vi "Process.vi"(8 "error in":errorcluster, 11 "Inst.Xeryon-Rotator":refnum<class "Inst.Xeryon-Rotator.lvclass">) -> (0 "error out":errorcluster, 3 "Inst.Xeryon-Rotator out":refnum<class "Inst.Xeryon-Rotator.lvclass">)   [LabVIEW 2019, in "Inst.Xeryon-Rotator.lvclass"]
doc: "---------------------------------------------------------------\nJKI State Machine Objects™\nhttp://jki.net/state-machine-objects/\nCopyright (C) 2005-2015, JKI <info@jki.net>\nALL RIGHTS RESERVED"
uses:
  Inst.Xeryon-Rotator.lvclass
  C:/Program Files (x86)/National Instruments/LabVIEW 2019/vi.lib/JKI/JKI SMO/SMO/SMO.lvclass
  C:/Program Files (x86)/National Instruments/LabVIEW 2019/user.lib/LevyLab/Instrument Framework/Instrument/Instrument.lvclass
  Typedefs/PrivateEvents--Inst.Xeryon-Rotator.MessageToProcess.ctl
  <userlib>/LevyLab/RemoteControl/RemoteControl/Typedefs/Message--Cluster.ctl
  <vilib>/JKI/JKI SMO/SMO/SMO.lvclass/SMO.ctl
  Inst.Xeryon-Rotator.lvclass/Inst.Xeryon-Rotator.ctl
  <userlib>/LevyLab/Instrument Framework/Instrument Types/Cryostat/Typedefs/setAngle--cluster.ctl
  Typedefs/Inst.Xeryon-Rotator.ScanState--Enum.ctl
  cbce47eb-2e04-4774-9aae-1c3eb2914706.vi
  f3e0a8c3-f545-4415-8120-73ea4d9772d3.vi
  828899be-930a-4dca-b584-bfe75166f4b0.vi
  bd7500a4-fca6-4b1e-8595-4df63a7e1bab.vi
  <vilib>/JKI/JKI SMO/SMO/Private/ReftoDVR--SMO.vi
  f3e0a8c3-f545-4415-8120-73ea4d9772d3.vi/fb9ef9f7-99d0-4ee5-81e5-6076cd542a2f.vi
  f3e0a8c3-f545-4415-8120-73ea4d9772d3.vi/df923573-e8f3-4648-a92f-bb60dda59a34.vi
  828899be-930a-4dca-b584-bfe75166f4b0.vi/24a7be02-affa-44f0-9bee-c77722484ac6.vi
  828899be-930a-4dca-b584-bfe75166f4b0.vi/9b5d2591-8431-4617-9ceb-7f0da0949f44.vi
  bd7500a4-fca6-4b1e-8595-4df63a7e1bab.vi/1d6531ba-9a80-485c-81e6-b1433e72d2e7.vi
  bd7500a4-fca6-4b1e-8595-4df63a7e1bab.vi/5f7f602e-e2b4-4f16-b1e8-66f0979bfccf.vi
  <vilib>/JDP Science/JSONtext/Variant to JSON Text.vi
  <vilib>/Utility/Data Type/Get Type Information.vi
  <vilib>/JDP Science/JSONtext/JSON text to Variant.vi
  <vilib>/JDP Science/JSONtext/LVClass Serializer/JSONtext LVClass Serializer.lvclass
  <userlib>/LevyLab/Instrument Framework/Instrument Types/Cryostat/Instrument.Cryostat.lvclass
  <userlib>/LevyLab/Instrument Framework/Instrument/Instrument.lvclass
  <userlib>/LevyLab/RemoteControl/RemoteControl/RemoteControl.lvclass
  <vilib>/JDP Science/JSONtext/JSONtext.lvlib
  <userlib>/LevyLab/Debug/Debug.lvlib
  <userlib>/LevyLab/Instrument Framework/Instrument/API/Instrument.sendMessageToProcess (variant).vi
  <vilib>/JKI/JKI SMO/SMO/SMO.lvclass
panel:
  out "Data":string
  out "Status":string
  out "State History":string
  # "Instrument.Xeryon-Rotator"
  # "Xeryon-Rotator"
  # "For instructions on how to use the JKI State Machine Objects, examples and video tutorials, visit:\nhttp://jki.net/state-machine-objects/\n\nJKI State Machine Objects™\nhttp://jki.net/state-machine-objects/\nCopyright (C) 2005-2015, JKI <info@jki.net>\nALL RIGHTS RESERVED"
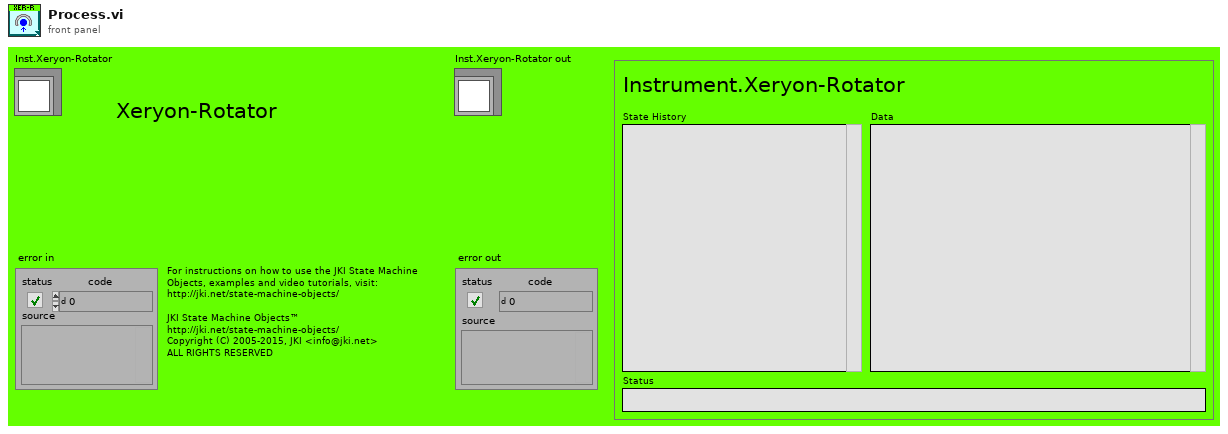
[diagram p1: front panel]
types:
  T1 = enum32{"invalid app kind", "Development System", "Run Time System", "Student Edition", "Embedded LabVIEW", "Evaluation", "Custom"}
  T2 = enum32{"Invalid", "Standard", "Closed", "Hidden", "Minimized", "Maximized"}
  T3 = typedef "Instrument.Cryostat.lvclass/setAngle--cluster.ctl" = cluster{"angle":dbl, "rate":dbl, "channel":i32}
  T4 = typedef "Inst.Xeryon-Rotator.lvclass/Inst.Xeryon-Rotator.ScanState--Enum.ctl" = enum16{"Scan Left", "Stop", "Scan Right", "Reset"}
  T5 = typedef "RemoteControl.lvlib/RemoteControl.lvclass/Message--Cluster.ctl" = cluster{"Command":string, "Data":variant, "ID":string, "error":errorcluster}
  T6 = typedef "Inst.Xeryon-Rotator.lvclass/PrivateEvents--Inst.Xeryon-Rotator.MessageToProcess.ctl" = cluster{"Message":T5}
  T7 = cluster{"Core":cluster{"Current VI Reference":refnum<vi>, "Close Panel on Exit?":bool, "Last Error":cluster{"error":errorcluster, "previous state":string, "remaining states":string}, "Shutdown?":bool}, "SelfRef":refnum<class "Inst.Xeryon-Rotator.lvclass">, "Running Step":i32, "sequence":string[], "MessageToProcess":T6}
  T8 = cluster{"Current VI Reference":refnum<vi>, "Close Panel on Exit?":bool, "Last Error":cluster{"error":errorcluster, "previous state":string, "remaining states":string}, "Shutdown?":bool}
  T9 = typedef "Debug.lvlib/Attribute.Debug.lvclass/DebugBehavior.ctl" = enum16{"Normal", "Debug"}
  T10 = typedef "SMO.lvclass/Protected Events.ctl" = cluster{"StopProcesses":refnum<user-event>, "AbortProcesses":refnum<user-event>, "Config Changed":refnum<user-event>, "Dependency":refnum<user-event>}
  T11 = cluster{"Encoder position [selected units]":dbl, "Desired Position [selected units]":dbl, "Status":string}
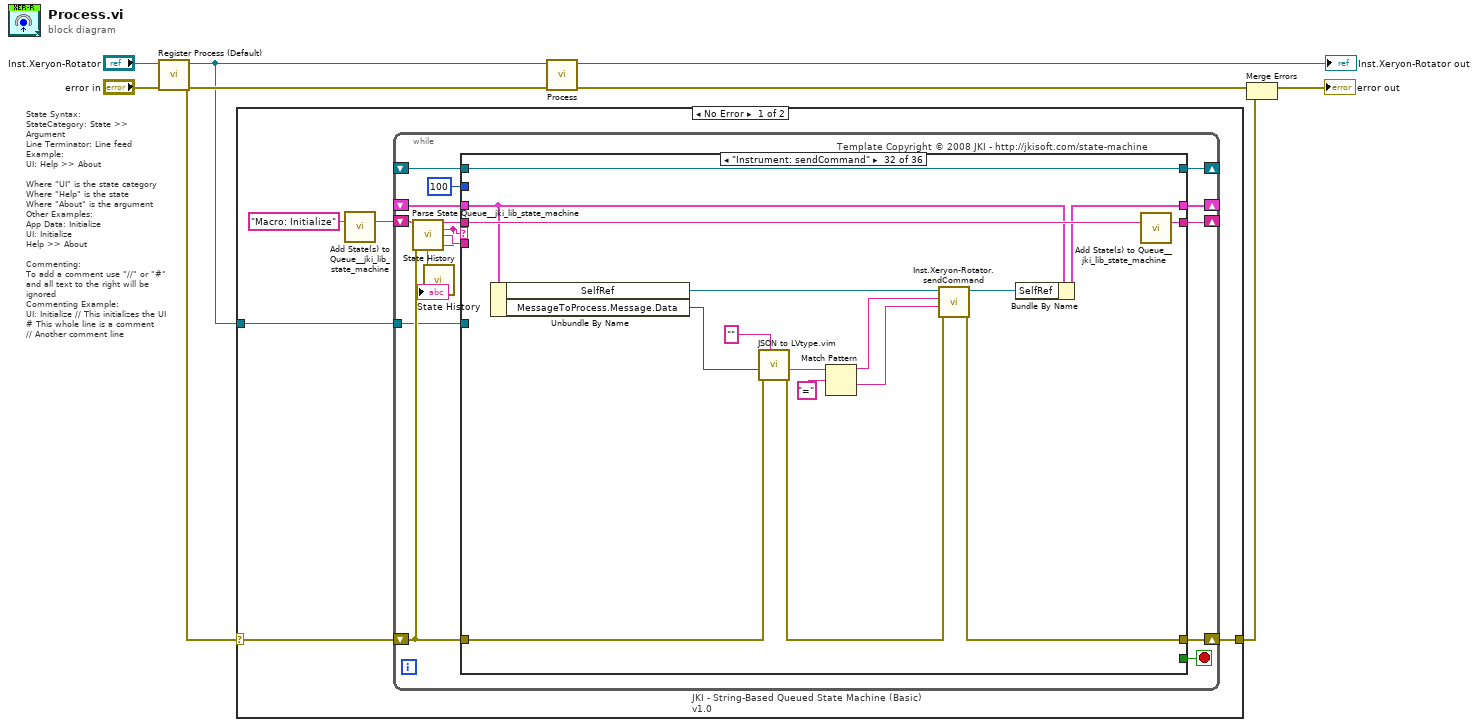
[diagram p0: block diagram]
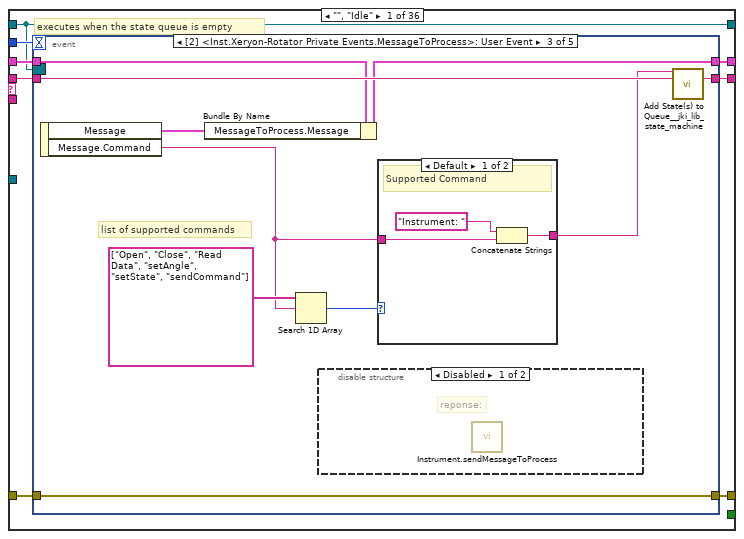
[diagram p2: hidden frame]
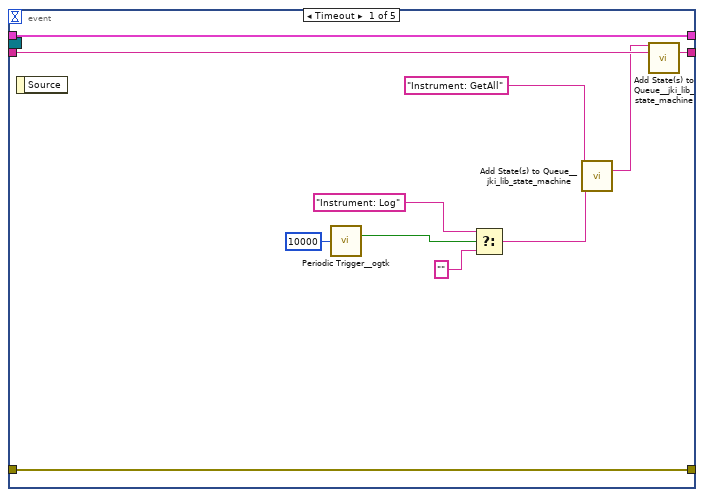
[diagram p3: hidden frame]
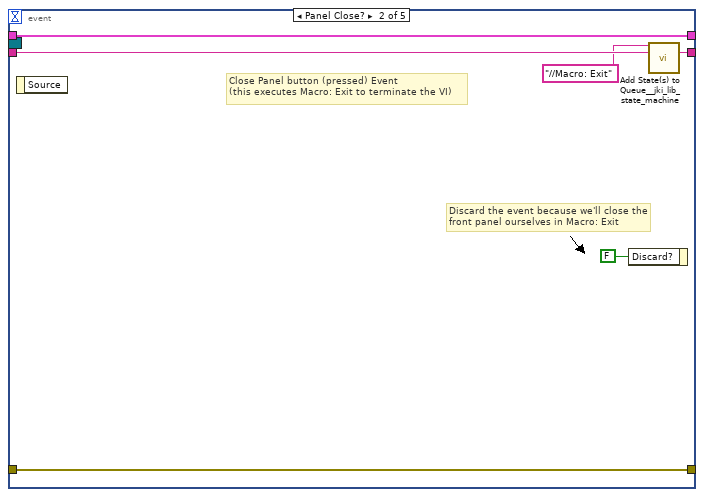
[diagram p4: hidden frame]
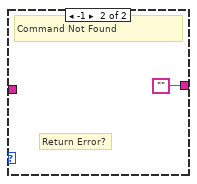
[diagram p6: hidden frame]
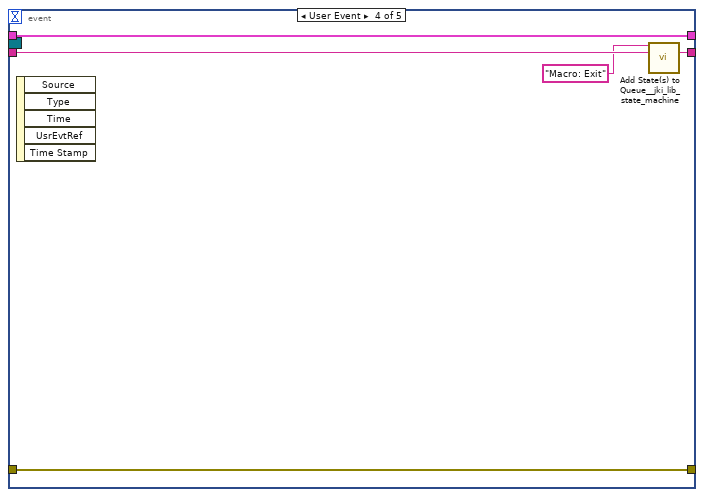
[diagram p7: hidden frame]
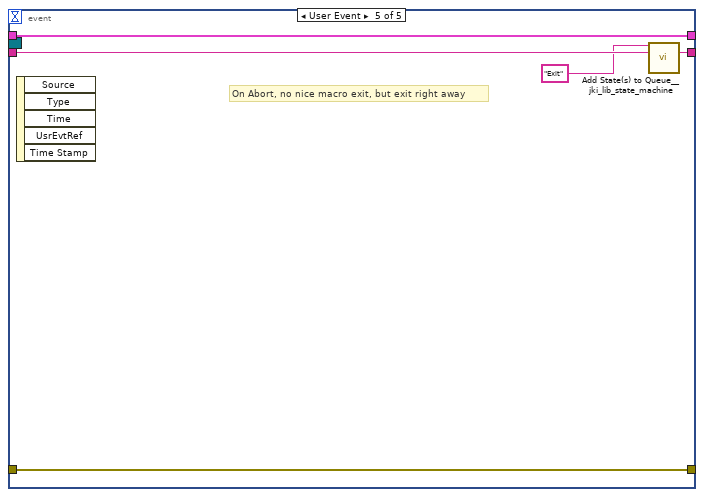
[diagram p8: hidden frame]
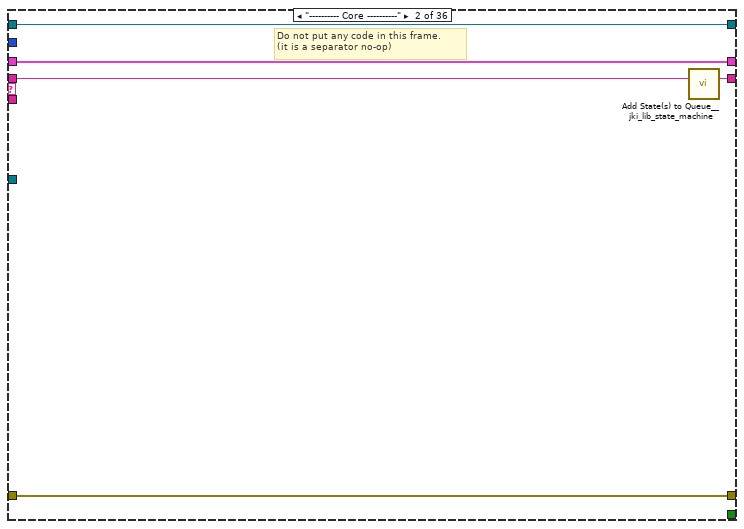
[diagram p9: hidden frame]
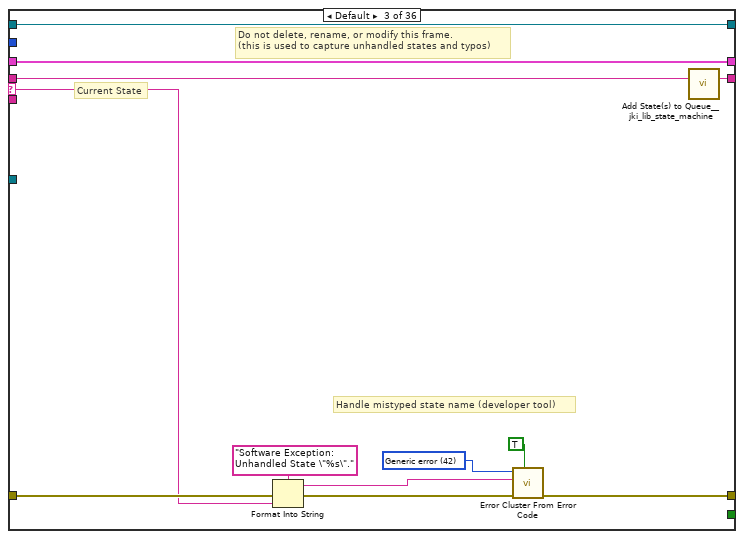
[diagram p10: hidden frame]
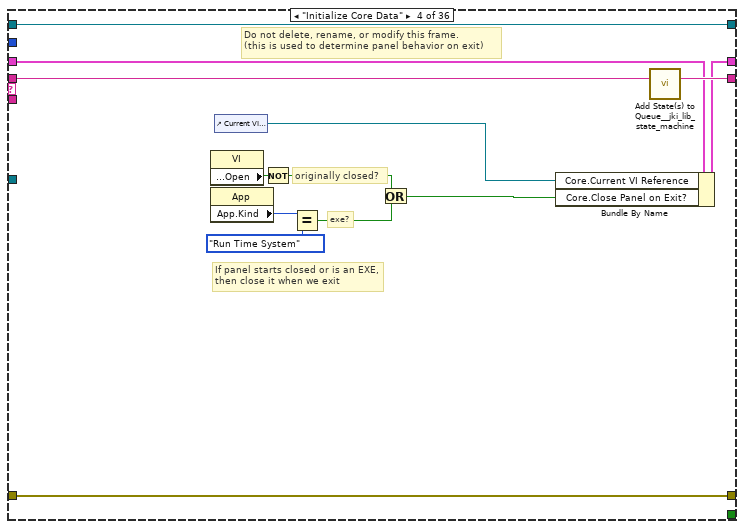
[diagram p11: hidden frame]
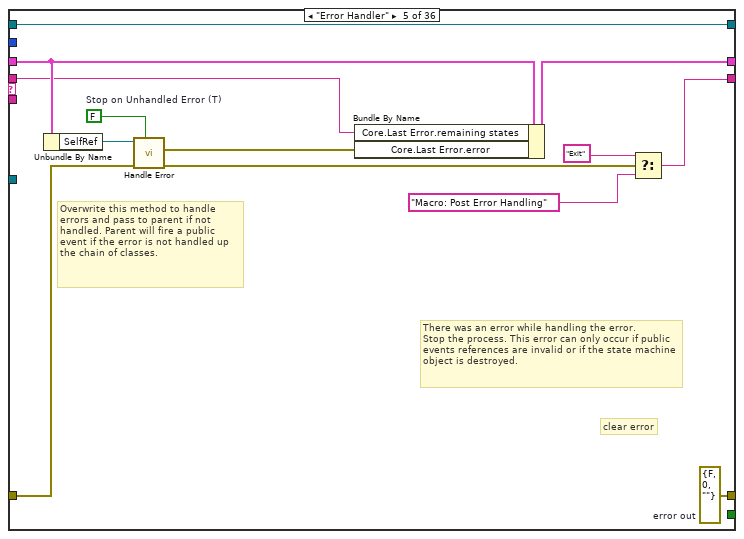
[diagram p12: hidden frame]
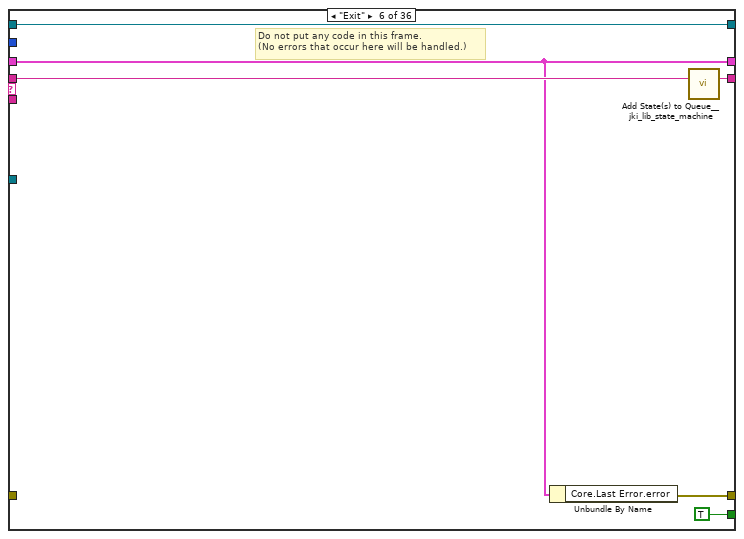
[diagram p13: hidden frame]
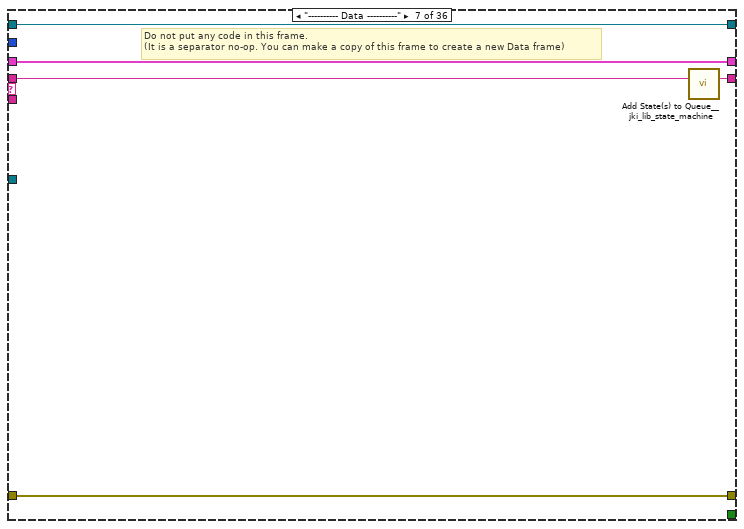
[diagram p14: hidden frame]
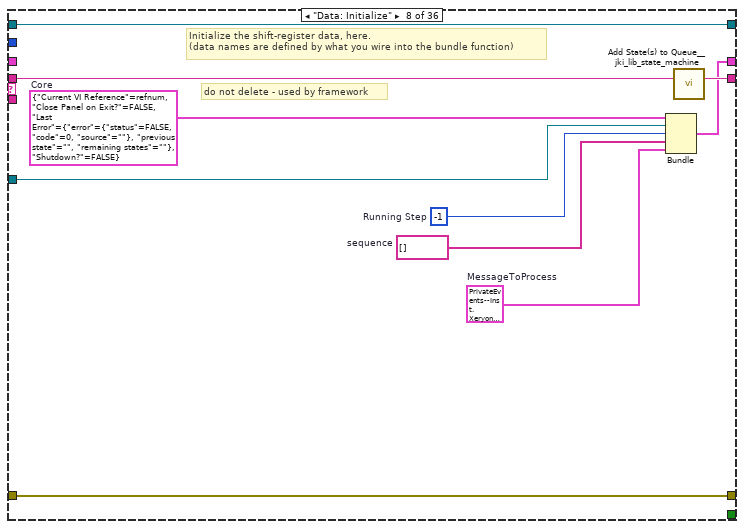
[diagram p15: hidden frame]
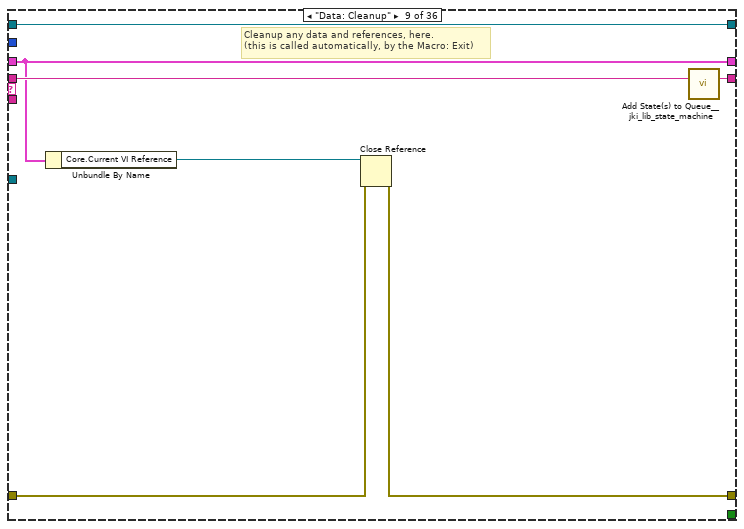
[diagram p16: hidden frame]
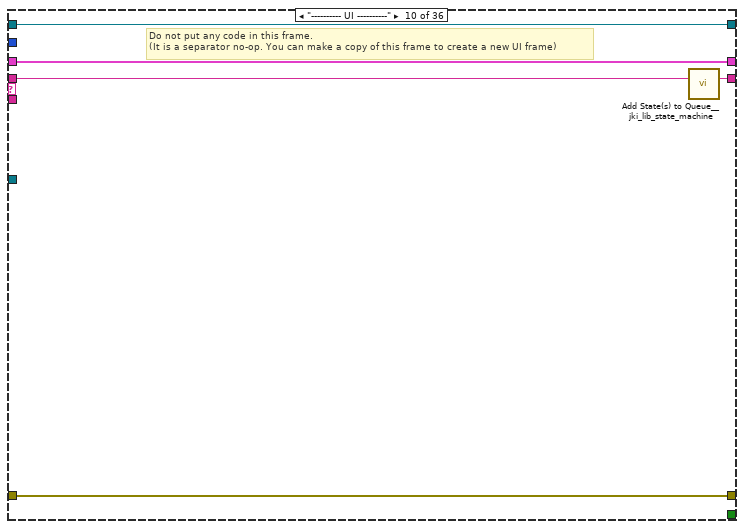
[diagram p17: hidden frame]
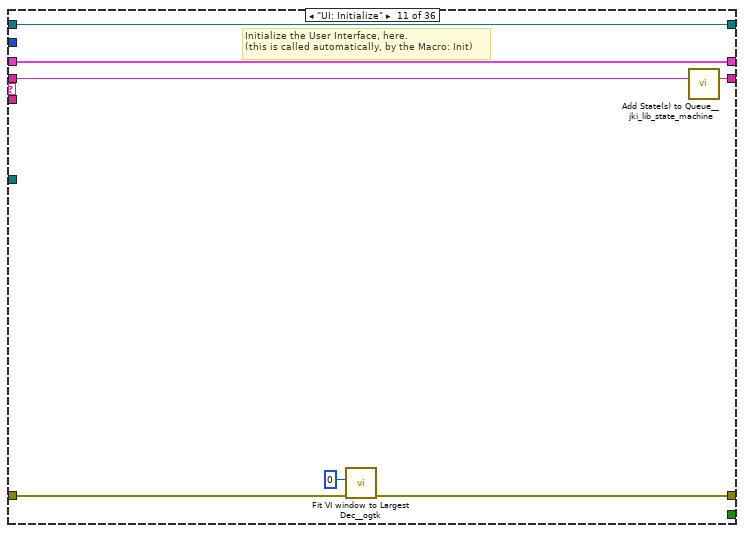
[diagram p18: hidden frame]
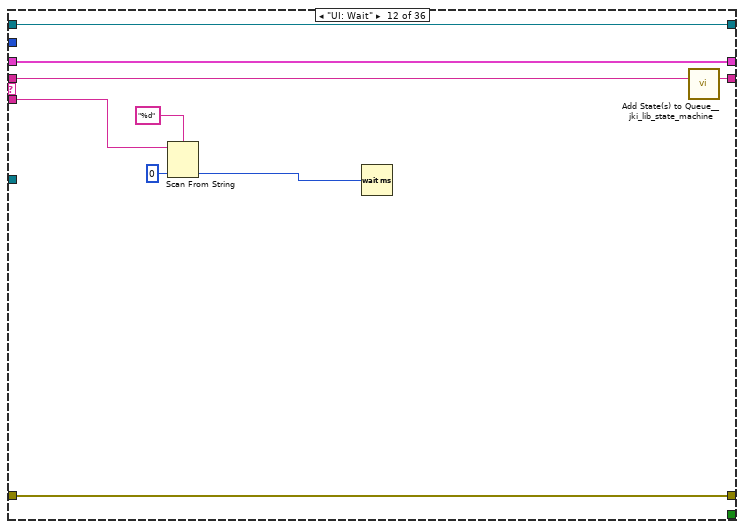
[diagram p19: hidden frame]
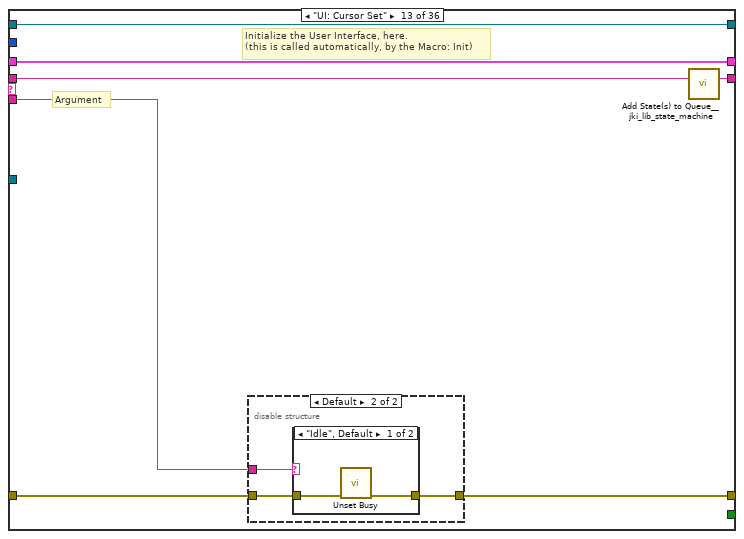
[diagram p20: hidden frame]
diagram:
  # "State Syntax:\nStateCategory: State >> Argument\nLine Terminator: Line feed\nExample:\nUI: Help >> About\n\nWhere \"UI\" is the state category\nWhere \"Help\" is the state\nWhere \"About\" is the argument\nOther Examples:\nApp Data: Initialize\nUI: Initialize\nHelp >> About\n\nCommenting:\nTo add a comment use \"//\" or \"#\" and all text to the right will be ignored\nCommenting Example:\nUI: Initialize // This initializes the UI\n# This whole line is a comment\n// Another comment line"
  n1 = call <vilib>:"Register Process (Default).vi"("error in (no error)"="error in", "SMO"="Inst.Xeryon-Rotator") -> ("error out"=w5:errorcluster, "SelfRef"=w4:refnum<class "Inst.Xeryon-Rotator.lvclass">)  [unwired: 8 in]
  n2 = case shown="No Error" w5 {
    selector: w5 -> [w10 w484]
    tunnel: w4 -> [w11 _]
    tunnel: [w9 w484] -> w1
    frame No Error {
      n3 = call <vilib>:"Add State(s) to Queue__jki_lib_state_machine.vi"("State(s) in (\"\")"="Macro: Initialize") -> ("States Out"=w13:string)  [unwired: 14 in]
      n4 = while "JKI - String-Based Queued State Machine (Basic) v1.0" {
        shift-right: [w22] -> _
        shift-left: _ -> [w21]
        shift-right: [w25] -> w9
        shift-left: w10 -> [w19]
        shift-right: [w24] -> _
        shift-left: w13 -> [w26]
        tunnel: w11 -> [w18]
        shift-right: [w17] -> _
        shift-left: _ -> [w16]
        stop <- w23 stop-if-true
        # "Template Copyright © 2008 JKI - http://jkisoft.com/state-machine"
        n5 = call <vilib>:"Parse State Queue__jki_lib_state_machine.vi"("State Queue"=w26, "Error In (no error)"=w19) -> ("Remaining States"=w28:string, "Current State"=w15:string, "Arguments"=w27:string)  [unwired: 11 in]
        n6 = call <userlib>:"State History.vi"("Current State"=w15) -> ("History"=→"State History":string)  [unwired: 10 in]
        n7 = case shown="\"Instrument: sendCommand\"" w15 {
          selector: w15 -> [_ _ w84 _ _ _ _ _ _ _ _ _ _ _ _ _ _ _ _ _ _ _ _ _ _ _ _ _ _ _ _ _ _ _ _ _]
          tunnel: w28 -> [w36 w82 w88 w107 w112 w126 w131 w141 w148 w153 w160 w169 w176 w192 w224 w233 w248 w265 w286 w303 w308 w319 w324 w337 w343 w350 w359 w368 w382 w408 w421 w437 w453 w458 w464 w483]
          tunnel: w27 -> [_ _ _ _ _ _ _ _ _ _ _ w161 w170 w186 _ _ _ _ _ _ _ _ _ _ _ _ _ _ _ _ _ _ _ _ w459 w467]
          tunnel: w21 -> [w34 w79 w86 w98 w116 w122 w128 _ w143 w150 w158 w166 w174 w188 w221 w230 w235 w255 w276 w290 w305 w316 w321 w330 w341 w345 w355 w364 w378 w404 w417 w433 w449 w454 w460 w473]
          tunnel: [w33 w80 w90 w104 w117 w121 w129 w133 w144 w151 w155 w167 w171 w189 w222 w225 w238 w263 w284 w292 w306 w310 w322 w333 w339 w347 w352 w361 w373 w403 w414 w426 w445 w455 w461 w475] -> w25
          tunnel: w19 -> [w32 w80 w89 w104 w118 _ w129 w133 w145 w151 w154 w167 w172 w190 w222 w225 w237 w263 w284 w292 w306 w311 w322 w327 w339 w347 w351 w360 w376 w392 w411 w431 w448 w455 w461 w469]
          tunnel: [w35 w81 w87 w106 w108 w125 w130 w140 w147 w152 w159 w168 w175 w191 w223 w232 w247 w264 w285 w302 w307 w318 w323 w336 w342 w349 w358 w367 w381 w407 w420 w436 w452 w457 w463 w482] -> w24
          tunnel: [_ _ _ _ _ TRUE _ _ _ _ _ _ _ _ _ _ _ _ _ _ _ _ _ _ _ _ _ _ _ _ _ _ _ _ _ _] -> w23
          tunnel: [w31 w79 w86 w105 w115 w122 w128 w139 w143 w150 w158 w166 w174 w188 w221 w230 w236 w256 w277 w287 w305 w316 w321 w330 w341 w346 w356 w365 w379 w405 w418 w434 w450 w454 w460 w472] -> w22
          tunnel: 100 ("Timeout") -> [w30 _ _ _ _ _ _ _ _ _ _ _ _ _ _ _ _ _ _ _ _ _ _ _ _ _ _ _ _ _ _ _ _ _ _ _]
          tunnel: w18 -> [_ _ _ _ _ _ _ w134 _ _ _ _ _ _ _ _ _ _ _ _ _ _ _ _ _ _ _ _ _ _ _ _ _ _ _ _]
          tunnel: [w29 w78 w83 w95 w120 w123 w127 w138 w142 w149 w157 w165 w173 w185 w220 w231 w246 w262 w283 w298 w304 w317 w320 w335 w340 w348 w357 w366 w380 w406 w419 w435 w451 w456 w462 w481] -> w17
          tunnel: w16 -> [w29 w78 w83 w95 w120 w123 w127 w138 w142 w149 w157 w165 w173 w185 w220 w231 w246 w262 w283 w298 w304 w317 w320 _ w340 w348 w357 w366 w380 w406 w419 w435 w451 w456 w462 w481]
          frame "", "Idle" {
            # "executes when the state queue is empty"
            n8 = event shown="[2] <Inst.Xeryon-Rotator Private Events.MessageToProcess>: User Event" {
              selector: w29 -> [_ _ _ _ _]
              dyn-events: _ -> [_ _ _ _ _]
              timeout: w30 -> [_ _ _ _ _]
              tunnel: w36 -> [w47 w53 w63 w72 w77]
              tunnel: [w46 w52 w62 w71 w76] -> w35
              tunnel: w34 -> [w44 w50 w55 w69 w74]
              tunnel: [w45 w51 w61 w70 w75] -> w33
              tunnel: w32 -> [w45 w51 w61 w70 w75]
              tunnel: [w44 w50 w56 w69 w74] -> w31
              event Timeout {
                n9 = event-data() -> ()  [unwired: 1 in, 1 out]
                n10 = call <userlib>:"Periodic Trigger__ogtk.vi"("time (ms)"=u32 10000) -> ("Triggered"=w41:bool)  [unwired: 12 in, 2 out]
                n11 = Select(t="Instrument: Log" ("State(s) in Front (\"\")"), s=w41, f="") -> (s? t:f=w40:string)
                n12 = call <vilib>:"Add State(s) to Queue__jki_lib_state_machine.vi"("State(s) in Front (\"\")"="Instrument: GetAll" ("State(s) in Front (\"\")"), "State(s) at Back (\"\")"=w40) -> ("States Out"=w38:string)  [unwired: 13 in]
                n13 = call <vilib>:"Add State(s) to Queue__jki_lib_state_machine.vi"("State(s) in Front (\"\")"=w38, "State(s) in (\"\")"=w47) -> ("States Out"=w46:string)  [unwired: 13 in]
              }
              event Panel Close? {
                # "Discard the event because we'll close the front panel ourselves in Macro: Exit"
                # "Close Panel button (pressed) Event\n(this executes Macro: Exit to terminate the VI)"
                n14 = event-data() -> ()  [unwired: 1 in, 1 out]
                n15 = event-data("Discard?"=FALSE) -> ()  [unwired: 1 in, 1 out]
                n16 = call <vilib>:"Add State(s) to Queue__jki_lib_state_machine.vi"("State(s) in Front (\"\")"="//Macro: Exit", "State(s) in (\"\")"=w53) -> ("States Out"=w52:string)  [unwired: 13 in]
              }
              event User Event {
                # "list of supported commands"
                n17 = event-data() -> ("Message"=w54:T5, "Message.Command"=w57:string)  [unwired: 1 in]
                n18 = Bundle By Name(cluster=w55, "MessageToProcess.Message"=w54) -> (w56:T7)
                n19 = Search 1D Array(1D array=string[] ["Open", "Close", "Read Data", "setAngle", "setState", "sendCommand"], element=w57) -> (index of element=w60:i32)  [unwired: 1 in]
                n20 = disable-structure shown="Disabled" {
                  frame Disabled {
                    # "reponse:"
                    n21 = call-poly <userlib>:"Instrument.sendMessageToProcess.vi"() -> ()  [unwired: 10 in, 2 out]
                  }
                  frame Enabled {
                  }
                }
                n22 = case shown="Default" w60 {
                  tunnel: [w66 "" ("Empty String Constant")] -> w58
                  tunnel: w57 -> [w65 _]
                  frame Default {
                    # "Supported Command"
                    n23 = Concatenate Strings("Instrument: ", w65) -> (w66:string)
                  }
                  frame -1 {
                    # "Return Error?"
                    # "Command Not Found"
                  }
                }
                n24 = call <vilib>:"Add State(s) to Queue__jki_lib_state_machine.vi"("State(s) in Front (\"\")"=w58, "State(s) in (\"\")"=w63) -> ("States Out"=w62:string)  [unwired: 13 in]
              }
              event User Event {
                n25 = event-data() -> ()  [unwired: 1 in, 5 out]
                n26 = call <vilib>:"Add State(s) to Queue__jki_lib_state_machine.vi"("State(s) in Front (\"\")"="Macro: Exit", "State(s) in (\"\")"=w72) -> ("States Out"=w71:string)  [unwired: 13 in]
              }
              event User Event {
                # "On Abort, no nice macro exit, but exit right away"
                n27 = event-data() -> ()  [unwired: 1 in, 5 out]
                n28 = call <vilib>:"Add State(s) to Queue__jki_lib_state_machine.vi"("State(s) in Front (\"\")"="Exit", "State(s) in (\"\")"=w77) -> ("States Out"=w76:string)  [unwired: 13 in]
              }
            }
          }
          frame "---------- Core ----------" {
            # "Do not put any code in this frame.\n(it is a separator no-op)"
            n29 = call <vilib>:"Add State(s) to Queue__jki_lib_state_machine.vi"("State(s) in (\"\")"=w82) -> ("States Out"=w81:string)  [unwired: 14 in]
          }
          frame Default {
            w93 = 42 items=["No error", "Argument error", "Memory is full", "Out of zone", "End of file", "File already open", "Generic file I/O error", "File not found", "File permission error", "Disk is full", "Duplicate path", "Too many files open", "System feature not enabled", "Resource file not found", "Cannot add resource", "Resource not found", "Image not found", "Image memory error", "Pen does not exist", "Config type invalid", "Config token not found", "Config parse error", "Config memory error", "Bad external code format", "Bad external code offset", "External code not present", "Null window", "Destroy window error", "Null menu", "Print aborted", "Bad print record", "Print driver error", "Windows error during printing", "Memory error during printing", "Print dialog error", "Generic print error", "Invalid device refnum", "Device not found", "Device parameter error", "Device unit error", "Cannot open device", "Device call aborted", "Generic error", "Cancelled by user", "Object ID too low", "Object ID too high", "Object not in heap", "Unknown heap", "Unknown object (invalid DefProc)", "Unknown object (DefProc not in table)", "Message out of range", "Invalid (null) method", "Unknown message", "Manager call not supported", "Bad address", "Network operation in progress", "Network operation timed out", "Connection is busy", "Network attribute not supported", "Network error", "Address in use", "System out of memory", "Connection aborted", "Connection refused", "Not connected", "Already connected", "Connection closed", "Initialization error (interapplication manager)", "Bad occurrence", "Wait on unbound occurrence handler", "Occurrence queue overflow", "Datalog type conflict", "Unused", "Unrecognized type (interapplication manager)", "Memory corrupt", "Failed to make temporary DLL", "Old CIN version", "Drag socket not found", "Failed to load drop-object", "Failed to register OLE object", "Failed to release OLE object", "Format specifier type mismatch", "Unknown format specifier", "Too few format specifiers", "Too many format specifiers", "Scan failed", "Newer CIN version", "Error converting to variant", "Runtime menu error", "Password tampered", "Variant attribute not found", "Incompatible variant data type", "Event data is not available", "Event Store is not present", "Occurrence is not found", "Event Queue is not created", "Event info is not available", "Refnum passed is NULL", "Error retrieving Class GUID", "Error retrieving CoClass GUID", "Error retrieving TypeLib GUID.", "Bad built application magic bytes.", "Specific driver is different from the specific driver associated with the Logical Name.", "There is no session opened to the class driver.", "Max Error", "MAX - Error with config objects", "MAX - Error loading configuration", "MAX - Group not supported"]
            # "Current State"
            # "Do not delete, rename, or modify this frame.\n(this is used to capture unhandled states and typos)"
            # "Handle mistyped state name (developer tool)"
            n30 = Format Into String(format string="Software Exception: Unhandled State \"%s\"." ("message"), error in=w89, w84) -> (resulting string=w92:string, error out=w91:errorcluster)  [unwired: 1 in]
            n31 = call <vilib>:"Error Cluster From Error Code.vi"("show call chain? (False)"=TRUE, "error in (no error)"=w91, "error message (\"\")"=w92, "error code (0)"=w93) -> ("error out"=w90:errorcluster)  [unwired: 5 in]
            n32 = call <vilib>:"Add State(s) to Queue__jki_lib_state_machine.vi"("State(s) in (\"\")"=w88) -> ("States Out"=w87:string)  [unwired: 14 in]
          }
          frame "Initialize Core Data" {
            # "Do not delete, rename, or modify this frame.\n(this is used to determine panel behavior on exit)"
            # "originally closed?"
            # "exe?"
            # "If panel starts closed or is an EXE, then close it when we exit"
            n33 = property class="VI"() -> ("Front Panel.Open"=w103:bool)  [unwired: 2 in, 2 out]
            n34 = property class="App"() -> ("App.Kind"=w102:T1)  [unwired: 2 in, 2 out]
            n35 = control-ref of="Current VI Reference"() -> (w96:refnum<vi>)
            n36 = Not(x=w103) -> (.not. x?=w100:bool)
            n37 = Equal?(x=w102, y=T1."Run Time System" ("Application:Kind")) -> (x = y?=w99:bool)
            n38 = Or(x=w100, y=w99) -> (x .or. y?=w97:bool)
            n39 = Bundle By Name(cluster=w98, "Core.Current VI Reference"=w96, "Core.Close Panel on Exit?"=w97) -> (w105:T7)
            n40 = call <vilib>:"Add State(s) to Queue__jki_lib_state_machine.vi"("State(s) in (\"\")"=w107) -> ("States Out"=w106:string)  [unwired: 14 in]
          }
          frame "Error Handler" {
            w113 = FALSE  # Stop on Unhandled Error (T)
            w117 = errorcluster {"status"=FALSE, "code"=0, "source"=""}  # error out
            # "clear error"
            # "There was an error while handling the error.\nStop the process. This error can only occur if public events references are invalid or if the state machine object is destroyed."
            # "Overwrite this method to handle errors and pass to parent if not handled. Parent will fire a public event if the error is not handled up the chain of classes."
            n41 = Unbundle By Name(w116) -> ("SelfRef"=w119:refnum<class "Inst.Xeryon-Rotator.lvclass">)
            n42 = call-dynamic "Handle Error.vi"("Stop on Unhandled Error (T)"=w113, "error in"=w118, "SMO"=w119) -> ("handling error"=w109:errorcluster, "Unhandled error"=w114:errorcluster)  [unwired: 6 in, 1 out]
            n43 = Bundle By Name(cluster=w116, "Core.Last Error.remaining states"=w112, "Core.Last Error.error"=w114) -> (w115:T7)
            n44 = Select(t="Exit", s=w109, f="Macro: Post Error Handling") -> (s? t:f=w108:string)
          }
          frame "Exit" {
            # "Do not put any code in this frame.\n(No errors that occur here will be handled.)"
            n45 = Unbundle By Name(w122) -> ("Core.Last Error.error"=w121:errorcluster)
            n46 = call <vilib>:"Add State(s) to Queue__jki_lib_state_machine.vi"("State(s) in (\"\")"=w126) -> ("States Out"=w125:string)  [unwired: 14 in]
          }
          frame "---------- Data ----------" {
            # "Do not put any code in this frame.\n(It is a separator no-op. You can make a copy of this frame to create a new Data frame)"
            n47 = call <vilib>:"Add State(s) to Queue__jki_lib_state_machine.vi"("State(s) in (\"\")"=w131) -> ("States Out"=w130:string)  [unwired: 14 in]
          }
          frame "Data: Initialize" {
            w132 = T6 {"Message"={"Command"="", "Data"=variant(string ""), "ID"="", "error"={"status"=FALSE, "code"=0, "source"=""}}}  # MessageToProcess
            w135 = string[] []  # sequence
            w136 = -1  # Running Step
            w137 = T8 {"Current VI Reference"=refnum, "Close Panel on Exit?"=FALSE, "Last Error"={"error"={"status"=FALSE, "code"=0, "source"=""}, "previous state"="", "remaining states"=""}, "Shutdown?"=FALSE}  # Core
            # "do not delete - used by framework"
            # "Initialize the shift-register data, here.\n(data names are defined by what you wire into the bundle function)"
            n48 = Bundle("Core"=w137, "SelfRef"=w134, "Running Step"=w136, "sequence"=w135, "MessageToProcess"=w132) -> (w139:T7)  [unwired: 1 in]
            n49 = call <vilib>:"Add State(s) to Queue__jki_lib_state_machine.vi"("State(s) in (\"\")"=w141) -> ("States Out"=w140:string)  [unwired: 14 in]
          }
          frame "Data: Cleanup" {
            # "Cleanup any data and references, here.\n(this is called automatically, by the Macro: Exit)"
            n50 = Unbundle By Name(w143) -> ("Core.Current VI Reference"=w146:refnum<vi>)
            n51 = Close Reference(reference=w146, error in (no error)=w145) -> (error out=w144:errorcluster)
            n52 = call <vilib>:"Add State(s) to Queue__jki_lib_state_machine.vi"("State(s) in (\"\")"=w148) -> ("States Out"=w147:string)  [unwired: 14 in]
          }
          frame "---------- UI ----------" {
            # "Do not put any code in this frame.\n(It is a separator no-op. You can make a copy of this frame to create a new UI frame)"
            n53 = call <vilib>:"Add State(s) to Queue__jki_lib_state_machine.vi"("State(s) in (\"\")"=w153) -> ("States Out"=w152:string)  [unwired: 14 in]
          }
          frame "UI: Initialize" {
            # "Initialize the User Interface, here.\n(this is called automatically, by the Macro: Init)"
            n54 = call <userlib>:"Fit VI window to Largest Dec__ogtk.vi"("error in (no error)"=w154, "border spacing (2 px)"=0) -> ("error out"=w155:errorcluster)  [unwired: 4 in, 1 out]
            n55 = call <vilib>:"Add State(s) to Queue__jki_lib_state_machine.vi"("State(s) in (\"\")"=w160) -> ("States Out"=w159:string)  [unwired: 14 in]
          }
          frame "UI: Wait" {
            n56 = Scan From String(format string="%d", input string=w161, default 1=u32 0 ("default value 1")) -> (output 1=w162:u32)  [unwired: 2 in, 3 out]
            n57 = Wait (ms)(milliseconds to wait=w162) -> ()  [unwired: 1 out]
            n58 = call <vilib>:"Add State(s) to Queue__jki_lib_state_machine.vi"("State(s) in (\"\")"=w169) -> ("States Out"=w168:string)  [unwired: 14 in]
          }
          frame "UI: Cursor Set" {
            # "Argument"
            # "Initialize the User Interface, here.\n(this is called automatically, by the Macro: Init)"
            n59 = disable-structure shown="Default" {
              disable-tunnel: w172 -> [w177 w180]
              disable-tunnel: [w177 w179] -> w171
              disable-tunnel: w170 -> [_ w178]
              frame condition #0 {
              }
              frame condition #1 (active) {
                n60 = case shown="\"Idle\", Default" w178 {
                  tunnel: w180 -> [w182 w184]
                  tunnel: [w181 w183] -> w179
                  frame "Idle", Default {
                    n61 = call <vilib>:"Unset Busy.vi"("error in (no error)"=w182) -> ("error out"=w181:errorcluster)  [unwired: 10 in]
                  }
                  frame "Busy" {
                    n62 = call <vilib>:"Set Busy.vi"("error in (no error)"=w184) -> ("error out"=w183:errorcluster)  [unwired: 9 in, 1 out]
                  }
                }
              }
            }
            n63 = call <vilib>:"Add State(s) to Queue__jki_lib_state_machine.vi"("State(s) in (\"\")"=w176) -> ("States Out"=w175:string)  [unwired: 14 in]
          }
          frame "UI: Front Panel State" {
            # "Argument"
            # "Set Front Panel Open or Closed\n(Usage: \"UI: Front Panel State >> Open|Close\")"
            n64 = Unbundle By Name(w188) -> ("Core.Current VI Reference"=w187:refnum<vi>)
            n65 = disable-structure shown="TARGET_TYPE==RT" {
              disable-tunnel: w190 -> [w196 w219]
              disable-tunnel: [w195 w219] -> w189
              disable-tunnel: w187 -> [w194 _]
              disable-tunnel: w186 -> [w193 _]
              frame condition #0 (active) {
                n66 = case shown="\"Close\"" w193 {
                  tunnel: w196 -> [w200 w213]
                  tunnel: [w202 w214] -> w195
                  tunnel: w194 -> [w201 w211]
                  frame "Open", Default {
                    n67 = property class="VI"(reference=w201, error in=w200) -> (reference out=w198:refnum<vi>, error out=w199:errorcluster, "FP.State"=w197:T2)
                    n68 = case shown="\"Closed\"" w197 {
                      tunnel: [w205 w208] -> w202
                      tunnel: w199 -> [w204 w208]
                      tunnel: w198 -> [w203 _]
                      frame "Closed" {
                        n69 = invoke class="VI" method="FP.Open"(reference=w203, error in=w204, "Activate"=TRUE, "State"=T2."Standard") -> (error out=w205:errorcluster)  [unwired: 1 in, 4 out]
                      }
                      frame Default {
                      }
                    }
                  }
                  frame "Close" {
                    n70 = property class="VI"(reference=w211, error in=w213) -> (reference out=w210:refnum<vi>, error out=w212:errorcluster, "FP.State"=w209:T2)
                    n71 = case shown="Default" w209 {
                      tunnel: [w215 w218] -> w214
                      tunnel: w212 -> [w215 w217]
                      tunnel: w210 -> [_ w216]
                      frame "Invalid", "Closed" {
                      }
                      frame Default {
                        n72 = invoke class="VI" method="FP.Close"(reference=w216, error in=w217) -> (error out=w218:errorcluster)  [unwired: 1 in, 2 out]
                      }
                    }
                  }
                }
              }
              frame condition #1 {
              }
            }
            n73 = call <vilib>:"Add State(s) to Queue__jki_lib_state_machine.vi"("State(s) in (\"\")"=w192) -> ("States Out"=w191:string)  [unwired: 14 in]
          }
          frame "---------- Macro ----------" {
            # "Do not put any code in this frame.\n(It is a separator no-op. You can make a copy of this frame to create a new Macro frame)"
            n74 = call <vilib>:"Add State(s) to Queue__jki_lib_state_machine.vi"("State(s) in (\"\")"=w224) -> ("States Out"=w223:string)  [unwired: 14 in]
          }
          frame "Macro: Initialize" {
            # "Initialization Macro\n(This is called once, when the VI starts)"
            n75 = call <vilib>:"Add State(s) to Queue__jki_lib_state_machine.vi"("State(s) in Front (\"\")"="Data: Initialize\nInitialize Core Data\nEvents: Register", "State(s) in (\"\")"="Process: Sync", "State(s) at Back (\"\")"="UI: Initialize\nUI: Front Panel State >> Close\nMacro: Debug\nInstrument: Open Hardware") -> ("States Out"=w228:string)  [unwired: 12 in]
            n76 = call <vilib>:"Add State(s) to Queue__jki_lib_state_machine.vi"("State(s) in Front (\"\")"=w228, "State(s) in (\"\")"=w233) -> ("States Out"=w232:string)  [unwired: 13 in]
          }
          frame "Macro: Debug" {
            # "exe?"
            # "If pane is an EXE, then close it when we exit"
            # "Macro: Debug\n(get debug behavior, determine UI and determine shutdown behavior)"
            n77 = Unbundle By Name(w235) -> ("Core.Close Panel on Exit?"=w240:bool, "SelfRef"=w245:refnum<class "Inst.Xeryon-Rotator.lvclass">)
            n78 = property class="App"() -> ("App.Kind"=w243:T1)  [unwired: 2 in, 2 out]
            n79 = Equal?(x=w243, y=T1."Run Time System" ("Application:Kind")) -> (x = y?=w239:bool)
            n80 = call <userlib>:"Get Debug Mode.vi"("error in (no error)"=w237, "SMO"=w245) -> ("error out"=w238:errorcluster, "Behavior"=w244:T9)  [unwired: 7 in, 1 out]
            n81 = case shown="\"Debug\"" w244 {
              tunnel: [w249 w251] -> w241
              tunnel: w240 -> [w249 _]
              tunnel: w239 -> [_ w253]
              tunnel: [_ "UI: Front Panel State >> Open\nUI: Wait >> 1000"] -> w234
              frame "Normal", Default {
                # "respect core.close"
              }
              frame "Debug" {
                # "keep panel open\nunless exe"
                n82 = Or(x=w253, y=FALSE) -> (x .or. y?=w251:bool)
              }
            }
            n83 = Bundle By Name(cluster=w235, "Core.Close Panel on Exit?"=w241) -> (w236:T7)
            n84 = call <vilib>:"Add State(s) to Queue__jki_lib_state_machine.vi"("State(s) in Front (\"\")"=w234, "State(s) in (\"\")"=w248) -> ("States Out"=w247:string)  [unwired: 13 in]
          }
          frame "Macro: Post Error Handling" {
            # "Clear Last Error?"
            n85 = Unbundle By Name(w255) -> ("Core.Last Error.remaining states"=w257:string, "Core.Shutdown?"=w258:bool)
            n86 = Unbundle By Name(w255) -> ("Core.Last Error.error"=w261:errorcluster)
            n87 = case shown="False" FALSE {
              tunnel: w261 -> [w269 _]
              tunnel: [w269 _] -> w260
              frame False {
              }
              frame True {
              }
            }
            n88 = case shown="True" w258 {
              tunnel: w257 -> [w266 w268]
              tunnel: [w266 w267] -> w254
              frame False {
                # "These are the remaining states (at the moment the error occured). States can be altered according to business logic."
                # "NOT SHUTTING DOWN"
              }
              frame True {
                # "Developer can decide to alter the states but should be aware that during the shutdown process, there are certain states that must be run for the SMO to properly shut itself (and this process) down. As such, one can add states to perform additional clean-ups, but should append the remaining state to be executed."
                # "SHUTTING DOWN"
                n89 = call <vilib>:"Add State(s) to Queue__jki_lib_state_machine.vi"("State(s) in (\"\")"=w268) -> ("States Out"=w267:string)  [unwired: 14 in]
              }
            }
            n90 = Bundle By Name(cluster=w255, "Core.Last Error.error"=w260) -> (w256:T7)
            n91 = call <vilib>:"Add State(s) to Queue__jki_lib_state_machine.vi"("State(s) in Front (\"\")"=w254, "State(s) in (\"\")"=w265) -> ("States Out"=w264:string)  [unwired: 13 in]
          }
          frame "Macro: Run Sequence" {
            # "0,1,2,3,4,"
            # "5"
            # "Do not put any code in this frame.\n(It is a separator no-op. You can make a copy of this frame to create a new Macro frame)"
            n92 = Unbundle By Name(w276) -> ("sequence"=w272:string[], "Running Step"=w270:i32)
            n93 = Array Size(array=w272) -> (size(s)=w282:i32)
            n94 = Index Array(array=w272, index=w270) -> (element=w271:string)
            n95 = Greater Or Equal?(x=w282, y=w270) -> (x >= y?=w274:bool)
            n96 = Select(t=-1 ("Running Step"), s=w274, f=w270) -> (s? t:f=w281:i32)
            n97 = Bundle By Name(cluster=w276, "Running Step"=w281) -> (w277:T7)
            n98 = Select(t="Sequence: Status >> ...", s=w274, f="Idle //Check Event Structure\nMacro: Run Sequence" ("State(s) at Back (\"\")")) -> (s? t:f=w273:string)
            n99 = call <vilib>:"Add State(s) to Queue__jki_lib_state_machine.vi"("State(s) in Front (\"\")"=w271, "State(s) at Back (\"\")"=w273) -> ("States Out"=w275:string)  [unwired: 13 in]
            n100 = call <vilib>:"Add State(s) to Queue__jki_lib_state_machine.vi"("State(s) in Front (\"\")"=w275, "State(s) in (\"\")"=w286) -> ("States Out"=w285:string)  [unwired: 13 in]
          }
          frame "Macro: Exit" {
            # "Exit Macro\n(This is called once, when the VI exits)"
            n101 = Unbundle By Name(w290) -> ("Core.Close Panel on Exit?"=w288:bool)
            n102 = Bundle By Name(cluster=w290, "Core.Shutdown?"=TRUE) -> (w287:T7)
            n103 = Select(t="UI: Front Panel State >> Close", s=w288, f="" ("Empty String Constant")) -> (s? t:f=w300:string)
            n104 = call <vilib>:"Add State(s) to Queue__jki_lib_state_machine.vi"("State(s) in Front (\"\")"="Data: Cleanup\nEvents: Unregister", "State(s) in (\"\")"="Process: Sync", "State(s) at Back (\"\")"="Exit") -> ("States Out"=w295:string)  [unwired: 12 in]
            n105 = call <vilib>:"Add State(s) to Queue__jki_lib_state_machine.vi"("State(s) in Front (\"\")"="Instrument: Close Hardware", "State(s) in (\"\")"=w300, "State(s) at Back (\"\")"=w295) -> ("States Out"=w299:string)  [unwired: 12 in]
            n106 = call <vilib>:"Add State(s) to Queue__jki_lib_state_machine.vi"("State(s) in Front (\"\")"=w299, "State(s) in (\"\")"=w303) -> ("States Out"=w302:string)  [unwired: 13 in]
          }
          frame "---------- Process ----------" {
            # "Template Separator\n(You can make a copy of, or modify, this frame)"
            n107 = call <vilib>:"Add State(s) to Queue__jki_lib_state_machine.vi"("State(s) in (\"\")"=w308) -> ("States Out"=w307:string)  [unwired: 14 in]
          }
          frame "Process: Sync" {
            n108 = Unbundle By Name(w316) -> ("SelfRef"=w312:refnum<class "Inst.Xeryon-Rotator.lvclass">)
            n109 = call <vilib>:"WaitOnProcessSync.vi"("error in (no error)"=w311, "SMO"=w312) -> ("error out"=w310:errorcluster, "Don't run?"=w315:bool)  [unwired: 7 in, 1 out]
            n110 = Select(t="Data: Cleanup\nEvents: Unregister\nExit", s=w315, f="" ("Empty String Constant")) -> (s? t:f=w309:string)
            n111 = call <vilib>:"Add State(s) to Queue__jki_lib_state_machine.vi"("State(s) in Front (\"\")"=w309, "State(s) in (\"\")"=w319) -> ("States Out"=w318:string)  [unwired: 13 in]
          }
          frame "---------- Events ----------" {
            # "Template Separator\n(You can make a copy of, or modify, this frame)"
            n112 = call <vilib>:"Add State(s) to Queue__jki_lib_state_machine.vi"("State(s) in (\"\")"=w324) -> ("States Out"=w323:string)  [unwired: 14 in]
          }
          frame "Events: Register" {
            n113 = Unbundle By Name(w330) -> ("SelfRef"=w331:refnum<class "Inst.Xeryon-Rotator.lvclass">)
            n114 = call <vilib>:"GetProtectedEvents.vi"("SMO"=w331) -> ("error out"=w329:errorcluster, "SMO Protected Events"=w334:T10, "SMO out"=w328:refnum<class "Inst.Xeryon-Rotator.lvclass">)  [unwired: 8 in]
            n115 = call "Inst.Xeryon-Rotator.GetPrivateEvents.vi"("Inst.Xeryon-Rotator in"=w328) -> ("error out"=w325:errorcluster, "Inst.Xeryon-Rotator Private Events"=w326:cluster{"MessageToProcess":refnum<user-event>})  [unwired: 8 in, 1 out]
            n116 = register-events(w334, w326) -> (reference out=w335:refnum<event-registration>, error out=w332:errorcluster)  [unwired: 2 in]
            n117 = Merge Errors(w332, w325, w329, w327) -> (w333:errorcluster)
            n118 = call <vilib>:"Add State(s) to Queue__jki_lib_state_machine.vi"("State(s) in (\"\")"=w337) -> ("States Out"=w336:string)  [unwired: 14 in]
          }
          frame "Events: Unregister" {
            n119 = Unregister For Events(event registration refnum=w340, error in=w339) -> (error out=w338:errorcluster)
            n120 = call <vilib>:"Clear Errors.vi"("error in (no error)"=w338) -> ()  [unwired: 5 in, 2 out]
            n121 = call <vilib>:"Add State(s) to Queue__jki_lib_state_machine.vi"("State(s) in (\"\")"=w343) -> ("States Out"=w342:string)  [unwired: 14 in]
          }
          frame "---------- Instrument ----------" {
            n122 = Unbundle By Name(w345) -> ("SelfRef"=w344:refnum<class "Inst.Xeryon-Rotator.lvclass">)
            n123 = Bundle By Name(cluster=w345, "SelfRef"=w344) -> (w346:T7)
            n124 = call <vilib>:"Add State(s) to Queue__jki_lib_state_machine.vi"("State(s) in (\"\")"=w350) -> ("States Out"=w349:string)  [unwired: 14 in]
          }
          frame "Instrument: Open Hardware" {
            n125 = Unbundle By Name(w355) -> ("SelfRef"=w354:refnum<class "Inst.Xeryon-Rotator.lvclass">)
            n126 = call-dynamic "Open Hardware.vi"("error in (no error)"=w351, "Inst.Xeryon-Rotator in"=w354) -> ("error out"=w352:errorcluster, "Inst.Xeryon-Rotator out"=w353:refnum<class "Inst.Xeryon-Rotator.lvclass">)  [unwired: 8 in]
            n127 = Bundle By Name(cluster=w355, "SelfRef"=w353) -> (w356:T7)
            n128 = call <vilib>:"Add State(s) to Queue__jki_lib_state_machine.vi"("State(s) in (\"\")"=w359) -> ("States Out"=w358:string)  [unwired: 14 in]
          }
          frame "Instrument: Close Hardware" {
            n129 = Unbundle By Name(w364) -> ("SelfRef"=w363:refnum<class "Inst.Xeryon-Rotator.lvclass">)
            n130 = call-dynamic "Close Hardware.vi"("error in (no error)"=w360, "Inst.Xeryon-Rotator in"=w363) -> ("error out"=w361:errorcluster, "Inst.Xeryon-Rotator out"=w362:refnum<class "Inst.Xeryon-Rotator.lvclass">)  [unwired: 8 in]
            n131 = Bundle By Name(cluster=w364, "SelfRef"=w362) -> (w365:T7)
            n132 = call <vilib>:"Add State(s) to Queue__jki_lib_state_machine.vi"("State(s) in (\"\")"=w368) -> ("States Out"=w367:string)  [unwired: 14 in]
          }
          frame "Instrument: GetAll" {
            # "communicate with\nhardware"
            n133 = Unbundle By Name(w378) -> ("SelfRef"=w377:refnum<class "Inst.Xeryon-Rotator.lvclass">, "MessageToProcess.Message.ID"=w369:string)
            n134 = call "Inst.Xeryon-Rotator.GetAllData.vi"("error in (no error)"=w376, "Inst.Xeryon-Rotator in"=w377) -> ("error out"=w372:errorcluster, "Data out"=w371:variant, "Inst.Xeryon-Rotator out"=w375:refnum<class "Inst.Xeryon-Rotator.lvclass">)  [unwired: 7 in]
            n135 = Empty String/Path?(string/path=w371) -> (empty?=w370:bool)
            n136 = case shown="False" w370 {
              tunnel: w375 -> [w387 w391]
              tunnel: [w386 w391] -> w374
              tunnel: [w384 w390] -> w373
              tunnel: w371 -> [w383 _]
              tunnel: w372 -> [w385 w390]
              tunnel: w369 -> [_ _]
              frame False {
                # "send data to\ninstrument:process.vi"
                n137 = call "To JSON Text.vim"("Anything"=w383) -> ("<JSON>"=w389:string)  [unwired: 9 in, 1 out]
                n138 = call <vilib>:"Pretty Print.vi"("JSON"=w389) -> ("<JSON>"=→"Data":string)  [unwired: 8 in, 2 out]
                n139 = call <userlib>:"setAllData.vi"("error in (no error)"=w385, "AllData"=w383, "Instrument in"=w387) -> ("error out"=w384:errorcluster, "Instrument out"=w386:refnum<class "Inst.Xeryon-Rotator.lvclass">)  [unwired: 7 in]
              }
              frame True {
              }
            }
            n140 = Bundle By Name(cluster=w378, "SelfRef"=w374) -> (w379:T7)
            n141 = call <vilib>:"Add State(s) to Queue__jki_lib_state_machine.vi"("State(s) in (\"\")"=w382) -> ("States Out"=w381:string)  [unwired: 14 in]
          }
          frame "Instrument: setAngle" {
            n142 = Unbundle By Name(w404) -> ("SelfRef"=w401:refnum<class "Inst.Xeryon-Rotator.lvclass">, "MessageToProcess.Message.Data"=w398:variant)
            n143 = call "JSON to LVtype.vim"("type"=T3 {"angle"=0.0, "rate"=0.0, "channel"=0} ("setAngle"), "error in (no error)"=w392, "JSON Data in"=w398) -> ("error out"=w393:errorcluster, "Data out"=w396:T3)  [unwired: 7 in]
            n144 = Unbundle By Name(w396) -> ("rate"=w395:dbl, "angle"=w394:dbl)
            n145 = call "Inst.Xeryon-Rotator.Set Speed.vi"("error in (no error)"=w393, "Rate (°/min)"=w395, "Inst.Xeryon-Rotator in"=w401) -> ("error out"=w399:errorcluster, "Inst.Xeryon-Rotator out"=w400:refnum<class "Inst.Xeryon-Rotator.lvclass">)  [unwired: 7 in]
            n146 = call "Inst.Xeryon-Rotator.Set Angle.vi"("error in (no error)"=w399, "Angle (°)"=w394, "Inst.Xeryon-Rotator in"=w400) -> ("error out"=w403:errorcluster, "Inst.Xeryon-Rotator out"=w402:refnum<class "Inst.Xeryon-Rotator.lvclass">)  [unwired: 7 in]
            n147 = Bundle By Name(cluster=w404, "SelfRef"=w402) -> (w405:T7)
            n148 = call <vilib>:"Add State(s) to Queue__jki_lib_state_machine.vi"("State(s) in (\"\")"=w408) -> ("States Out"=w407:string)  [unwired: 14 in]
          }
          frame "Instrument: setState" {
            n149 = Unbundle By Name(w417) -> ("SelfRef"=w416:refnum<class "Inst.Xeryon-Rotator.lvclass">, "MessageToProcess.Message.Data"=w413:variant)
            n150 = call "JSON to LVtype.vim"("type"=Inst.Xeryon-Rotator.ScanState--Enum."Stop" ("Scan State"), "error in (no error)"=w411, "JSON Data in"=w413) -> ("error out"=w412:errorcluster, "Data out"=w409:T4)  [unwired: 7 in]
            n151 = call "Inst.Xeryon-Rotator.Set State.vi"("error in (no error)"=w412, "Scan State"=w409, "Inst.Xeryon-Rotator in"=w416) -> ("error out"=w414:errorcluster, "Inst.Xeryon-Rotator out"=w415:refnum<class "Inst.Xeryon-Rotator.lvclass">)  [unwired: 7 in]
            n152 = Bundle By Name(cluster=w417, "SelfRef"=w415) -> (w418:T7)
            n153 = call <vilib>:"Add State(s) to Queue__jki_lib_state_machine.vi"("State(s) in (\"\")"=w421) -> ("States Out"=w420:string)  [unwired: 14 in]
          }
          frame "Instrument: sendCommand" {
            n154 = Unbundle By Name(w433) -> ("SelfRef"=w429:refnum<class "Inst.Xeryon-Rotator.lvclass">, "MessageToProcess.Message.Data"=w432:variant)
            n155 = call "JSON to LVtype.vim"("type"="", "error in (no error)"=w431, "JSON Data in"=w432) -> ("error out"=w427:errorcluster, "Data out"=w424:string)  [unwired: 7 in]
            n156 = Match Pattern(string=w424, regular expression="=") -> (before substring=w423:string, after substring=w422:string)  [unwired: 1 in, 2 out]
            n157 = call "Inst.Xeryon-Rotator.sendCommand.vi"("error in (no error)"=w427, "Value"=w422, "Command"=w423, "Inst.Xeryon-Rotator in"=w429) -> ("error out"=w426:errorcluster, "Inst.Xeryon-Rotator out"=w428:refnum<class "Inst.Xeryon-Rotator.lvclass">)  [unwired: 6 in]
            n158 = Bundle By Name(cluster=w433, "SelfRef"=w428) -> (w434:T7)
            n159 = call <vilib>:"Add State(s) to Queue__jki_lib_state_machine.vi"("State(s) in (\"\")"=w437) -> ("States Out"=w436:string)  [unwired: 14 in]
          }
          frame "Instrument: Log" {
            n160 = Unbundle By Name(w449) -> ("SelfRef"=w438:refnum<class "Inst.Xeryon-Rotator.lvclass">)
            n161 = call-dynamic "Get SMO Database Paths.vi"("error in (no error)"=w448, "Inst.Xeryon-Rotator in"=w438) -> ("error out"=w446:errorcluster, "Paths"=w447:string, "Inst.Xeryon-Rotator out"=w440:refnum<class "Inst.Xeryon-Rotator.lvclass">)  [unwired: 7 in]
            n162 = Unbundle By Name(w440) -> ("Encoder position [selected units]"=w444:dbl, "Desired Position [selected units]"=w442:dbl, "Status"=w441:string)
            n163 = Bundle("Encoder position [selected units]"=w444, "Desired Position [selected units]"=w442, "Status"=w441) -> (w443:T11)  [unwired: 1 in]
            n164 = call <userlib>:"Instrument.logToDatabase.vi"("error in (no error)"=w446, "Data"=w443, "Paths"=w447, "Instrument"=w440) -> ("error out"=w445:errorcluster, "Instrument out"=w439:refnum<class "Inst.Xeryon-Rotator.lvclass">)  [unwired: 6 in]
            n165 = Bundle By Name(cluster=w449, "SelfRef"=w439) -> (w450:T7)
            n166 = call <vilib>:"Add State(s) to Queue__jki_lib_state_machine.vi"("State(s) in (\"\")"=w453) -> ("States Out"=w452:string)  [unwired: 14 in]
          }
          frame "---------- Sequence ----------" {
            n167 = call <vilib>:"Add State(s) to Queue__jki_lib_state_machine.vi"("State(s) in (\"\")"=w458) -> ("States Out"=w457:string)  [unwired: 14 in]
          }
          frame "Sequence: Status" {
            # "Sequence: Status\n(Use this frame to pass the status to the UI, this VI's UI, etc)"
            n168 = call <vilib>:"Add State(s) to Queue__jki_lib_state_machine.vi"("State(s) in (\"\")"=w464) -> ("States Out"=w463:string)  [unwired: 14 in]
            "Status" <- w459
          }
          frame "Sequence: Wait" {
            # "Sequence: Wait\n(Non-Blocking Wait)"
            # "F = repeat this state. wait\nT = go to next state. don't wait"
            n169 = Unbundle By Name(w473) -> ("Running Step"=w466:i32)
            n170 = call <userlib>:"Wait Logic.vi"("error in (no error)"=w469, "Time"=w467) -> ("error out"=w468:errorcluster, "Status String"=w465:string, "Trigger"=w470:bool)  [unwired: 6 in, 1 out]
            n171 = Increment(x=w466) -> (x+1=w480:i32)
            n172 = Select(t=w480, s=w470, f=w466) -> (s? t:f=w471:i32)
            n173 = Select(t=u32 0, s=w470, f=u32 100 ("milliseconds to wait")) -> (s? t:f=w477:u32)
            n174 = call <userlib>:"Wait (ms)__ogtk.vi"("error in (no error)"=w468, "milliseconds to wait"=w477) -> ("error out"=w475:errorcluster)  [unwired: 8 in, 1 out]
            n175 = Bundle By Name(cluster=w473, "Running Step"=w471) -> (w472:T7)
            n176 = call <vilib>:"Build State String with Arguments__JKI_lib_State_Machine.vi"("Arguments (\"\")"=w465, "State"="Sequence: Status") -> ("State with Arguments"=w474:string)  [unwired: 4 in]
            n177 = call <vilib>:"Add State(s) to Queue__jki_lib_state_machine.vi"("State(s) in Front (\"\")"=w474, "State(s) in (\"\")"=w483) -> ("States Out"=w482:string)  [unwired: 13 in]
          }
        }
      }
    }
    frame Error {
    }
  }
  n178 = call-parent "Process.vi"("error in"=w5, "Instrument"=w4) -> ("error out"=w2:errorcluster, "Instrument out"=→"Inst.Xeryon-Rotator out":refnum<class "Inst.Xeryon-Rotator.lvclass">)  [unwired: 8 in]
  n179 = Merge Errors(w2, w1) -> (→"error out":errorcluster)
